vi "Cleanup Arrays.vi"(9 "Time axis":dbl[](array[numeric]), 10 "Array to Clean":dbl[](array[numeric])) -> (1 "Time Values":dbl[](array[numeric]), 2 "Cleaned Array":dbl[][](array[numeric]))   [LabVIEW 2014, in "Melody Extraction.lvlib"]
uses:
  Melody Extraction.lvlib
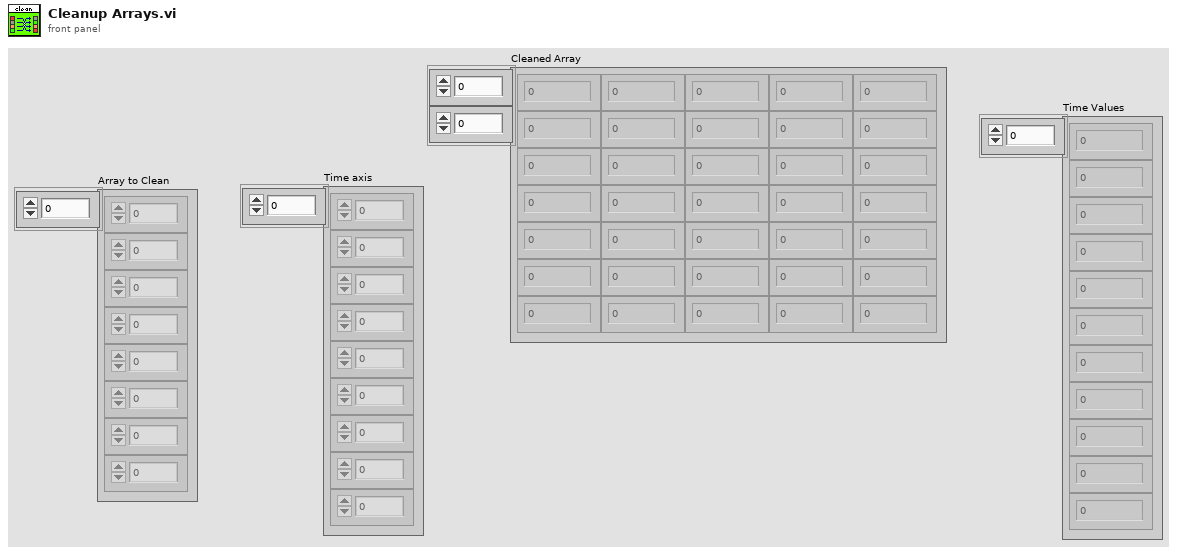
[diagram p1: front panel]
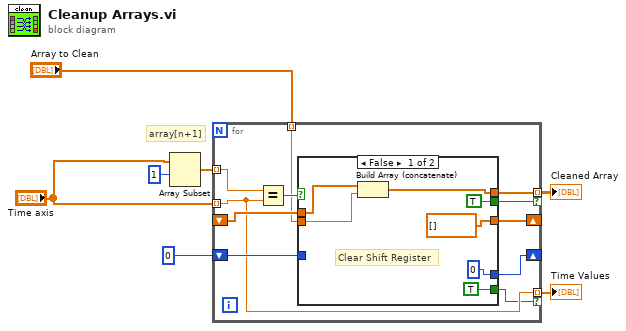
[diagram p0: block diagram]
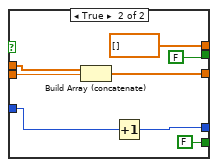
[diagram p2: hidden frame]
diagram:
  # "array[n+1]"
  n1 = Array Subset(array="Time axis", index=1) -> (w5:dbl[])  [unwired: 1 in]
  n2 = for {
    tunnel: "Time axis" -> [w9] mode=indexing
    tunnel: w5 -> [w18] mode=indexing
    shift-right: [w15] -> _
    shift-left: 0 -> [w16]
    shift-right: [w14] -> _
    shift-left: _ -> [w13]
    tunnel: [w12] -> w3 mode=indexing if=w11
    tunnel: "Array to Clean" -> [w10] mode=indexing
    tunnel: [w9] -> w2 mode=indexing if=w8
    n3 = Equal?(x=w18, y=w9) -> (x = y?=w17:bool)
    n4 = case shown="False" w17 {
      tunnel: w16 -> [_ w33]
      tunnel: [0 w32] -> w15
      tunnel: w10 -> [w19 w31]
      tunnel: [dbl[] [] w30] -> w14
      tunnel: w13 -> [w21 w29]
      tunnel: [w20 dbl[] []] -> w12
      tunnel: [TRUE FALSE] -> w11
      tunnel: [TRUE FALSE] -> w8
      frame False {
        # "Clear Shift Register"
        n5 = Build Array (concatenate)(w21, w19) -> (w20:dbl[])
      }
      frame True {
        n6 = Build Array (concatenate)(w29, w31) -> (w30:dbl[])
        n7 = Increment(x=w33) -> (x+1=w32:i32)
      }
    }
  }
  "Cleaned Array" <- w3
  "Time Values" <- w2
